vi "AlazarGetBoardBySystemId.vi"(3 "error in (no error)":errorcluster, 4 "Board ID":u32=1, 5 "System ID":u32=1) -> (0 "error out":errorcluster, 1 "Return Code":u32, 2 "Handle":u64)   [LabVIEW 2018]
doc: "Get a handle to a board in a board system where the board system is specified its system identifier and the board by its board identifier within the board system."
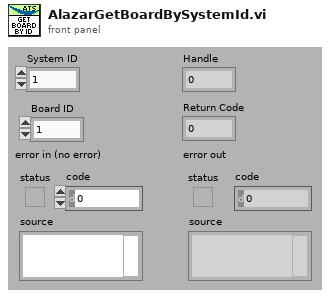
[diagram p1: front panel]
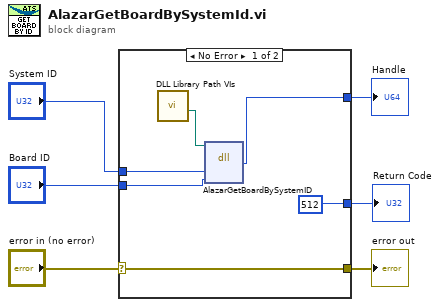
[diagram p0: block diagram]
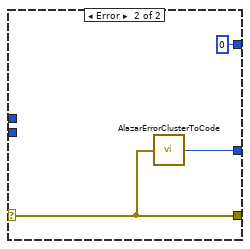
[diagram p2: hidden frame]
diagram:
  n1 = case shown="No Error" "error in (no error)" {
    selector: "error in (no error)" -> [w9 w15]
    tunnel: [w9 w15] -> w5
    tunnel: "System ID" -> [w12 _]
    tunnel: [w10 u32 0] -> w3
    tunnel: "Board ID" -> [w11 _]
    tunnel: [512 w14] -> w1
    frame No Error {
      n2 = call "DLL Library Path VIs.vi"() -> ("Alazar"=w7:path)  [unwired: 4 in, 7 out]
      n3 = dll-call lib="C:/Project/SerialSectOCT - FFT GPU/SerialSectOCT/Labview Software/Hardware Mfg/AlazarTech SDK/ATSApi.dll" fn="AlazarGetBoardBySystemID"(path in=w7, "systemID"=w12, "boardID"=w11) -> ("return type"=w10:u64)  [unwired: 4 in, 2 out]
    }
    frame Error {
      n4 = call "AlazarErrorClusterToCode.vi"("error in (no error)"=w15) -> ("Error Code"=w14:u32)
    }
  }
  "Handle" <- w3
  "error out" <- w5
  "Return Code" <- w1
